vi "Element position on graph.vi"(6 "Check Element":bool, 7 "Spectrum":refnum<vi>, 8 "List":string[](array[string]), 9 "String":string, 10 "List Elements in":string[](array[string]), 11 "Elements Position Peaks in":dbl[][](array[numeric])) -> (2 "List Elements out":string[](array[string]), 3 "Element Position Peaks out":dbl[][](array[numeric]))   [LabVIEW 2023]
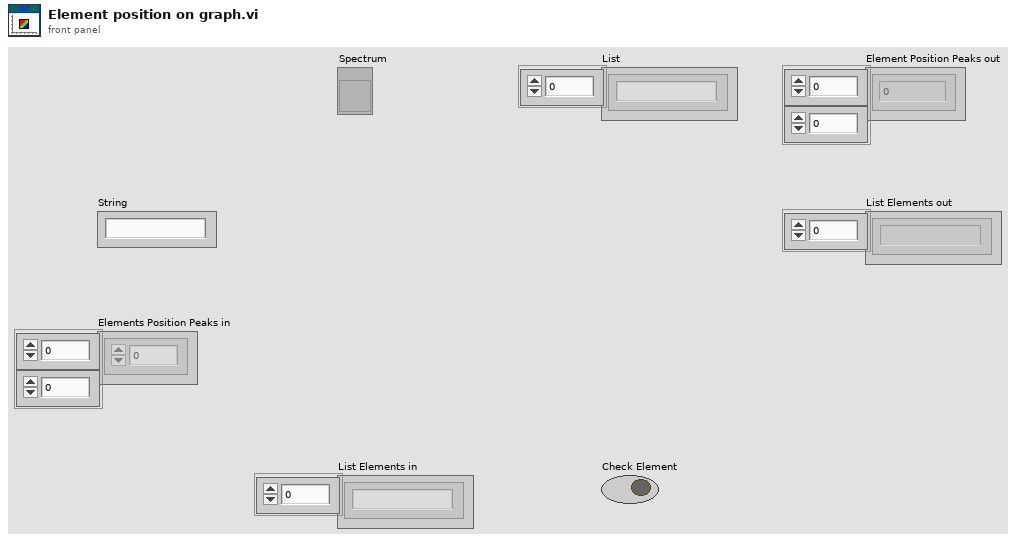
[diagram p1: front panel]
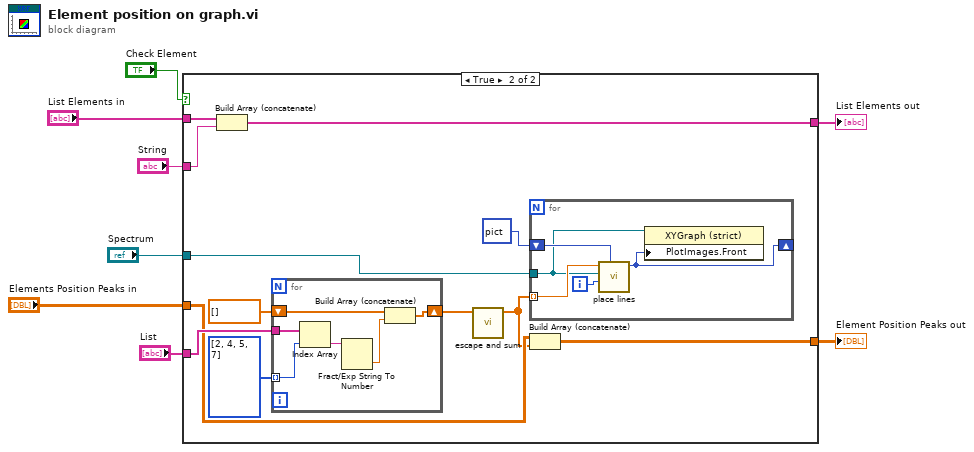
[diagram p0: block diagram]
diagram:
  n1 = case shown="True" "Check Element" {
    tunnel: "List" -> [_ w22]
    tunnel: "Elements Position Peaks in" -> [w10 w19]
    tunnel: [w10 w18] -> w4
    tunnel: "String" -> [_ w16]
    tunnel: [w9 w15] -> w7
    tunnel: "List Elements in" -> [w9 w14]
    tunnel: "Spectrum" -> [_ w11]
    frame False {
    }
    frame True {
      n2 = Build Array (concatenate)(w14, w16) -> (w15:string[])
      n3 = for {
        tunnel: w22 -> [w33]
        tunnel: i32[] [2, 4, 5, 7] -> [w32] mode=indexing
        shift-right: [w31] -> w17
        shift-left: dbl[] [] -> [w30]
        n4 = Index Array(array=w33, index=w32) -> (element=w29:string)
        n5 = Fract/Exp String To Number(string=w29) -> (number=w28:dbl)  [unwired: 3 in, 1 out]
        n6 = Build Array (concatenate)(w30, w28) -> (w31:dbl[])
      }
      n7 = call "escape and sum.vi"("List in"=w17) -> ("List Out"=w13:dbl[])  [unwired: 10 in]
      n8 = for {
        tunnel: w13 -> [w27] mode=indexing
        tunnel: w11 -> [w23]
        shift-right: [w25] -> _
        shift-left: picture data[5B] ("line to place") -> [w24]
        i -> [w26]
        n9 = call "place lines.vi"("picture in"=w24, "line"=w26, "Graph"=w23, "Energy"=w27) -> ("line to place"=w25:picture)  [unwired: 7 in]
        n10 = property on="Property Node" class="XYGraph (strict)"(reference=w23, "PlotImages.Front"=w25) -> ()  [unwired: 1 in, 2 out]
      }
      n11 = Build Array (concatenate)(w19, w13) -> (w18:dbl[][])
    }
  }
  "List Elements out" <- w7
  "Element Position Peaks out" <- w4
